vi "Measurement Logic.vi"() -> ()   [LabVIEW 2024, in "Device Power Sequencer.lvlib"]
uses:
  Device Power Sequencer.lvlib
  <vilib>/Plug-In SDKs/Measurements/Measure Call Context/Measure Call Context.lvclass
  Measurement Configuration.ctl
  controls/Source Mode.ctl
  controls/Sense Mode.ctl
  controls/Relative To.ctl
  controls/Transient Response.ctl
  controls/Power line frequency.ctl
  Measurement Results.ctl
  coreLogic/devicePowerSequencerCoreLogic.lvlib
panel:
  out "measurement results":T1
  in  "measurement configuration":T2={"Quick Power Down"=TRUE, "Pin Name"=["", ""], "Source Mode"=[32, 33], "Start Value"=[64.0, 65.0], "Target Value"=[0.0, 0.0], "Compliance Limit"=[-32.0, -33.0], "Sense Mode"=[0, 0], "Default Ramp Rate"=[FALSE, FALSE], "Ramp Rate"=[-64.0, -65.0], "Start Delay"=[], "Relative To"=[], "Transient Response"=[], "Data Capture"=FALSE, "Power line frequency"=1} {"Relative To" items=["Power sequence start", "Previous source start", "Previous source end"]; "Power line frequency" items=["Rabbit", "Gopher", "Badger"]; "Start Value" format="%#_6p"; "Transient Response" items=["Slow", "Normal", "Fast"]; "Sense Mode" items=["Local Sense", "Remote Sense"]; "Target Value" format="%#_6p"; "Source Mode" items=["DC Voltage", "DC Current"]; "Start Delay" format="%#_6p"; "Compliance Limit" format="%#_6p"; "Ramp Rate" format="%#_6p"}
  out "measure call context out":refnum<class "Measure Call Context.lvclass">
  in  "measure call context in":refnum<class "Measure Call Context.lvclass">
  out "error out":errorcluster
  in  "error in":errorcluster
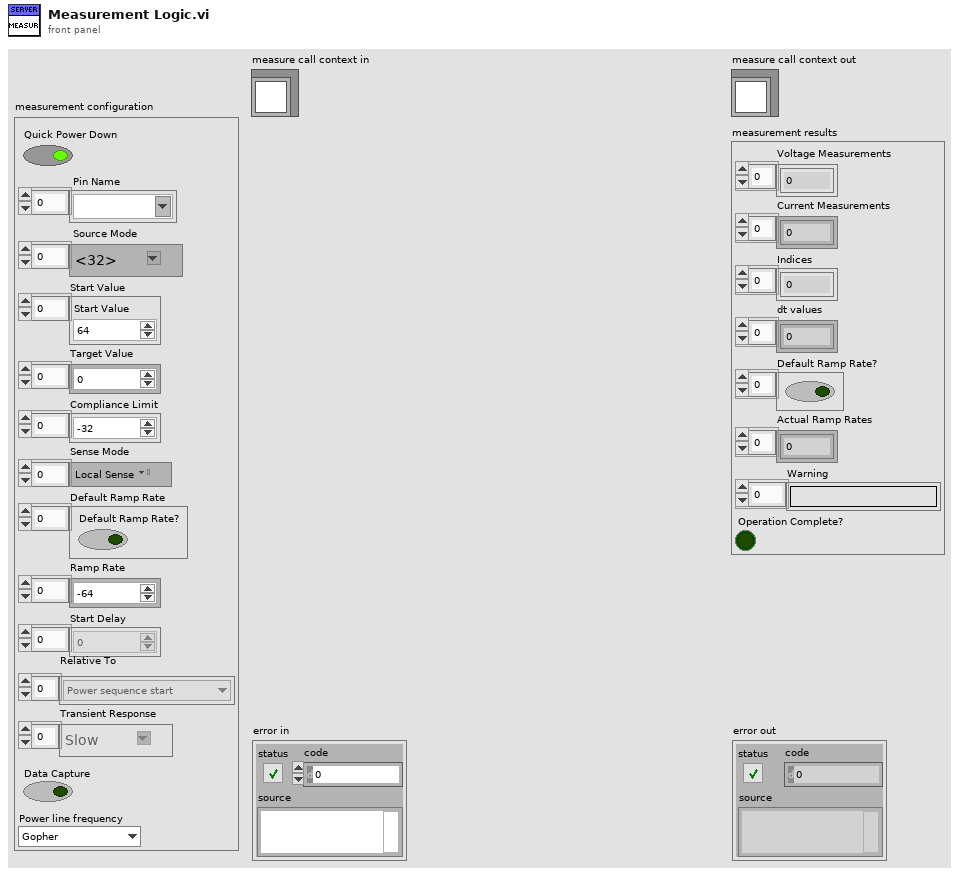
[diagram p1: front panel]
types:
  T1 = typedef "Device Power Sequencer.lvlib/Measurement Results.ctl" = cluster{"Voltage Measurements":dbl[], "Current Measurements":dbl[], "Indices":i32[], "dt values":dbl[], "Default Ramp Rate?":bool[], "Actual Ramp Rates":dbl[], "Warning":string[], "Operation Complete?":bool}
  T2 = typedef "Device Power Sequencer.lvlib/Measurement Configuration.ctl" = cluster{"Quick Power Down":bool, "Pin Name":string[], "Source Mode":T3[], "Start Value":dbl[], "Target Value":dbl[], "Compliance Limit":dbl[], "Sense Mode":T4[], "Default Ramp Rate":bool[], "Ramp Rate":dbl[], "Start Delay":dbl[], "Relative To":T5[], "Transient Response":T6[], "Data Capture":bool, "Power line frequency":T7}
  T3 = typedef "Device Power Sequencer.lvlib/Source Mode.ctl" = i32
  T4 = typedef "Device Power Sequencer.lvlib/Sense Mode.ctl" = i32
  T5 = typedef "Device Power Sequencer.lvlib/Relative To.ctl" = u32
  T6 = typedef "Device Power Sequencer.lvlib/Transient Response.ctl" = i32
  T7 = typedef "Device Power Sequencer.lvlib/Power line frequency.ctl" = u32
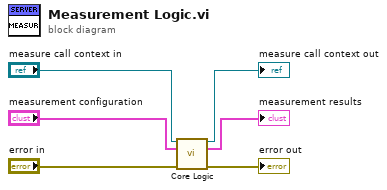
[diagram p0: block diagram]
diagram:
  n1 = call "Core Logic.vi"("Measurement Context In"="measure call context in", "Measurement Configuration"="measurement configuration", "error in"="error in") -> ("Measurement Context Out"=→"measure call context out":refnum<class "Measure Call Context.lvclass">, "Measurement Results"=→"measurement results":T1, "error out"=→"error out":errorcluster)  [unwired: 10 in]
